vi "SSL Read.vi"(7 "Buffer Size":i32=1024, 8 "Error In":errorcluster) -> (0 "Error Out":errorcluster, 2 "Message Read":string)   [LabVIEW 2012, in "SSL Lib.lvlib"]
doc: "VI Function: This VI reads the data from client over the SSL stream.\n\nVI Version: 1.0\n\nVI Author: Runjhun Agarwal"
uses:
  <userlib>/SSL Library/SSL Lib.lvlib
  <userlib>/SSL Library/Controls/Ref.ctl
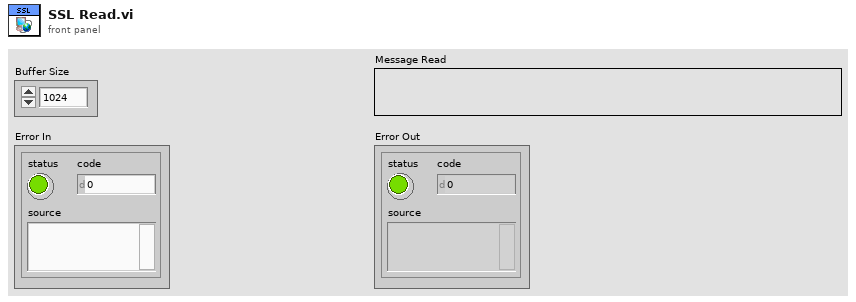
[diagram p1: front panel]
types:
  T1 = typedef "Ref.ctl" = enum16{"Update Ref", "Read Ref", "Close Ref"}
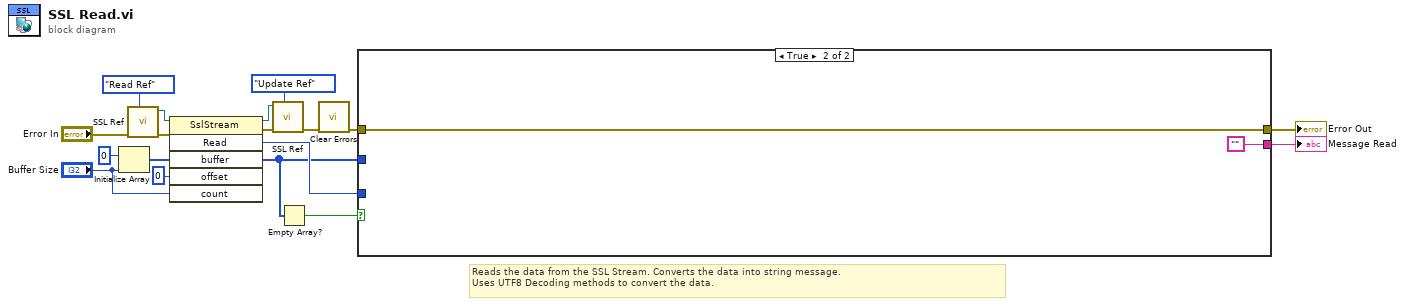
[diagram p0: block diagram]
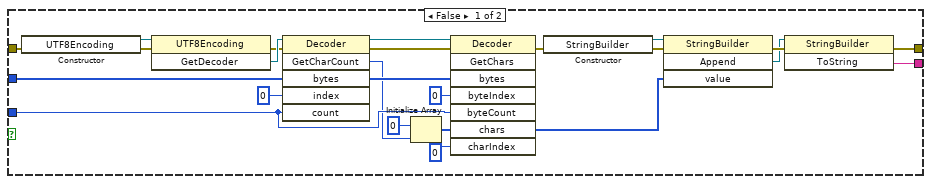
[diagram p2: hidden frame]
diagram:
  # "Reads the data from the SSL Stream. Converts the data into string message.\nUses UTF8 Decoding methods to convert the data."
  n1 = Initialize Array(u8 0 ("element"), "Buffer Size") -> (w17:u8[])
  n2 = call <userlib>:"SSL Ref.vi"("Action"=Ref."Read Ref", "Error In"="Error In") -> ("Error Out"=w10:errorcluster, "SSL Stream"=w9:refnum<k24>)  [unwired: 8 in]
  n3 = invoke class="SslStream" method="Read"(reference=w9, error in=w10, "buffer"=w17, "offset"=0, "count"="Buffer Size") -> (reference out=w7:refnum<k24>, error out=w6:errorcluster, "Read"=w15:i32, "buffer"=w2:u8[])  [unwired: 1 in, 2 out]
  n4 = call <userlib>:"SSL Ref.vi"("Action"=Ref."Update Ref", "Error In"=w6, "SSL Stream"=w7) -> ("Error Out"=w4:errorcluster)  [unwired: 7 in, 1 out]
  n5 = Empty Array?(array=w2) -> (empty?=w1:bool)
  n6 = call <vilib>:"Clear Errors.vi"("error in (no error)"=w4) -> ("error out"=w3:errorcluster)  [unwired: 6 in]
  n7 = case shown="True" w1 {
    tunnel: w15 -> [w34 _]
    tunnel: [w28 ""] -> w14
    tunnel: [w21 w44] -> w12
    tunnel: w3 -> [w20 w44]
    tunnel: w2 -> [w19 _]
    frame False {
      n8 = constructor class="UTF8Encoding"(error in=w20) -> (reference out=w39:refnum<k24>, error out=w40:errorcluster)  [unwired: 2 in, 1 out]
      n9 = invoke class="UTF8Encoding" method="GetDecoder"(reference=w39, error in=w40) -> (error out=w41:errorcluster, "GetDecoder"=w42:refnum<k24>)  [unwired: 1 in, 1 out]
      n10 = invoke class="Decoder" method="GetCharCount"(reference=w42, error in=w41, "bytes"=w19, "index"=0, "count"=w34) -> (reference out=w37:refnum<k24>, error out=w36:errorcluster, "GetCharCount"=w26:i32, "bytes"=w35:u8[])  [unwired: 1 in, 2 out]
      n11 = Initialize Array(u16 0 ("element"), w26) -> (w24:u16[])
      n12 = invoke class="Decoder" method="GetChars"(reference=w37, error in=w36, "bytes"=w35, "byteIndex"=0, "byteCount"=w34, "chars"=w24, "charIndex"=0 ("byteIndex")) -> (error out=w29:errorcluster, "chars"=w22:u16[])  [unwired: 1 in, 6 out]
      n13 = constructor class="StringBuilder"(error in=w29) -> (reference out=w30:refnum<k24>, error out=w33:errorcluster)  [unwired: 2 in, 1 out]
      n14 = invoke class="StringBuilder" method="Append"(reference=w30, error in=w33, "value"=w22) -> (error out=w32:errorcluster, "Append"=w31:refnum<k24>)  [unwired: 1 in, 2 out]
      n15 = invoke class="StringBuilder" method="ToString"(reference=w31, error in=w32) -> (error out=w21:errorcluster, "ToString"=w28:string)  [unwired: 1 in, 1 out]
    }
    frame True {
    }
  }
  "Message Read" <- w14
  "Error Out" <- w12
